vi "Default Settings.vi"() -> ()   [LabVIEW 2017]
uses:
  CTLs/Template Frame.ctl
  CTLs/Text Format.ctl
panel:
  out "font width":i16[](array[numeric])=[2, 2, 4, 6, 4, 4, 5, 2, 3, 3, 4, 4, 2, 3, 2, 3, 4, 3, 4, 4, 4, 4, 4, 4, 4, 4, 2, 2, 4, 3, 4, 3, 4, 4, 4, 4, 4, 3, 3, 4, 4, 2, 3, 4, 3, 4, 4, 4, 4, 4, 4, 4, 4, 4, 4, 4, 4, 4, 4, 3, 3, 3, 4, 4, 3, 4, 4, 4, 4, 3, 3, 4, 4, 2, 3, 4, 3, 4, 4, 4, 4, 4, 4, 4, 4, 4, 4, 4, 4, 4, 4, 4, 3, 4, 5]
  out "font":picture[](array[picture])=[bytes[60], bytes[60], bytes[90], bytes[120], bytes[90], bytes[90], bytes[105], bytes[60], bytes[75], bytes[75], bytes[90], bytes[90], bytes[60], bytes[75], bytes[60], bytes[75], bytes[90], bytes[75], bytes[90], bytes[90], bytes[90], bytes[90], bytes[90], bytes[90], bytes[90], bytes[90], bytes[60], bytes[60], bytes[90], bytes[75], bytes[90], bytes[75], bytes[90], bytes[90], bytes[90], bytes[90], bytes[90], bytes[75], bytes[75], bytes[90], bytes[90], bytes[60], bytes[75], bytes[90], bytes[75], bytes[90], bytes[90], bytes[90], bytes[90], bytes[90], bytes[90], bytes[90], bytes[90], bytes[90], bytes[90], bytes[90], bytes[90], bytes[90], bytes[90], bytes[75], bytes[75], bytes[75], bytes[90], bytes[90], bytes[75], bytes[90], bytes[90], bytes[90], bytes[90], bytes[75], bytes[75], bytes[90], bytes[90], bytes[60], bytes[75], bytes[90], bytes[75], bytes[90], bytes[90], bytes[90], bytes[90], bytes[90], bytes[90], bytes[90], bytes[90], bytes[90], bytes[90], bytes[90], bytes[90], bytes[90], bytes[90], bytes[90], bytes[75], bytes[90], bytes[105]]
  in  "text format":T1
  in  "template frame":T2=enum."compact lib"
  in  "color":string="black"
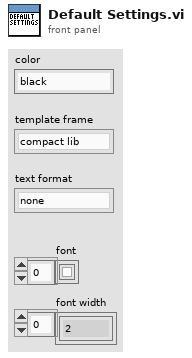
[diagram p1: front panel]
types:
  T1 = typedef "Text Format.ctl" = enum16{"none"}
  T2 = typedef "Template Frame.ctl" = enum16{"none", "compact lib"}
diagram:
